vi "PAQmem_WriteOne.vi"(7 "Carry":bool, 8 "error in (no error)":errorcluster, 10 "StoreDatagram":T1 {"Time" format="%#.2f"; "status" format="%x"; "min" format="%.2f"; "max" format="%.2f"; "data" format="%.2f"}, 11 "PAQ-memory in":refnum<class "PAQ-memory.lvclass">) -> (0 "error out":errorcluster, 1 "Last":i32, 2 "Prev":i32, 3 "PAQ-memory out":refnum<class "PAQ-memory.lvclass">)   [LabVIEW 2020, in "Sgraph_lib_V1.lvlib" / "PAQ-memory.lvclass"]
doc: "PAQ memory action: write one sample (of multiple TAGs)\n\nThis VI writes one array of TAGs to the computer memory DVR element"
uses:
  PAQ-memory.lvclass
  controls/MemStoreDatagram.ctl
  PAQ-memory.lvclass/PAQ-memory.ctl
  FAMM.lvclass
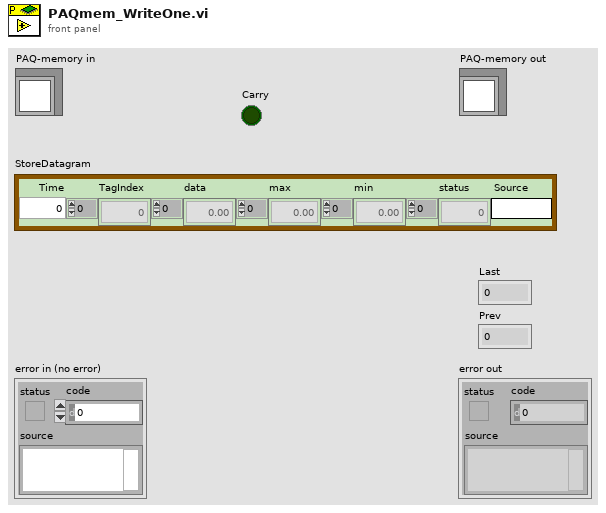
[diagram p1: front panel]
types:
  T1 = typedef "Sgraph_lib_V1.lvlib/FAMM.lvclass/MemStoreDatagram.ctl" = cluster{"Time":dbl, "TagIndex":i32[], "data":dbl[], "max":dbl[], "min":dbl[], "status":u32[], "Source":string}
  T2 = cluster{"source":refnum<data-value>, "status":refnum<data-value>, "data":refnum<data-value>, "max":refnum<data-value>, "min":refnum<data-value>}[]
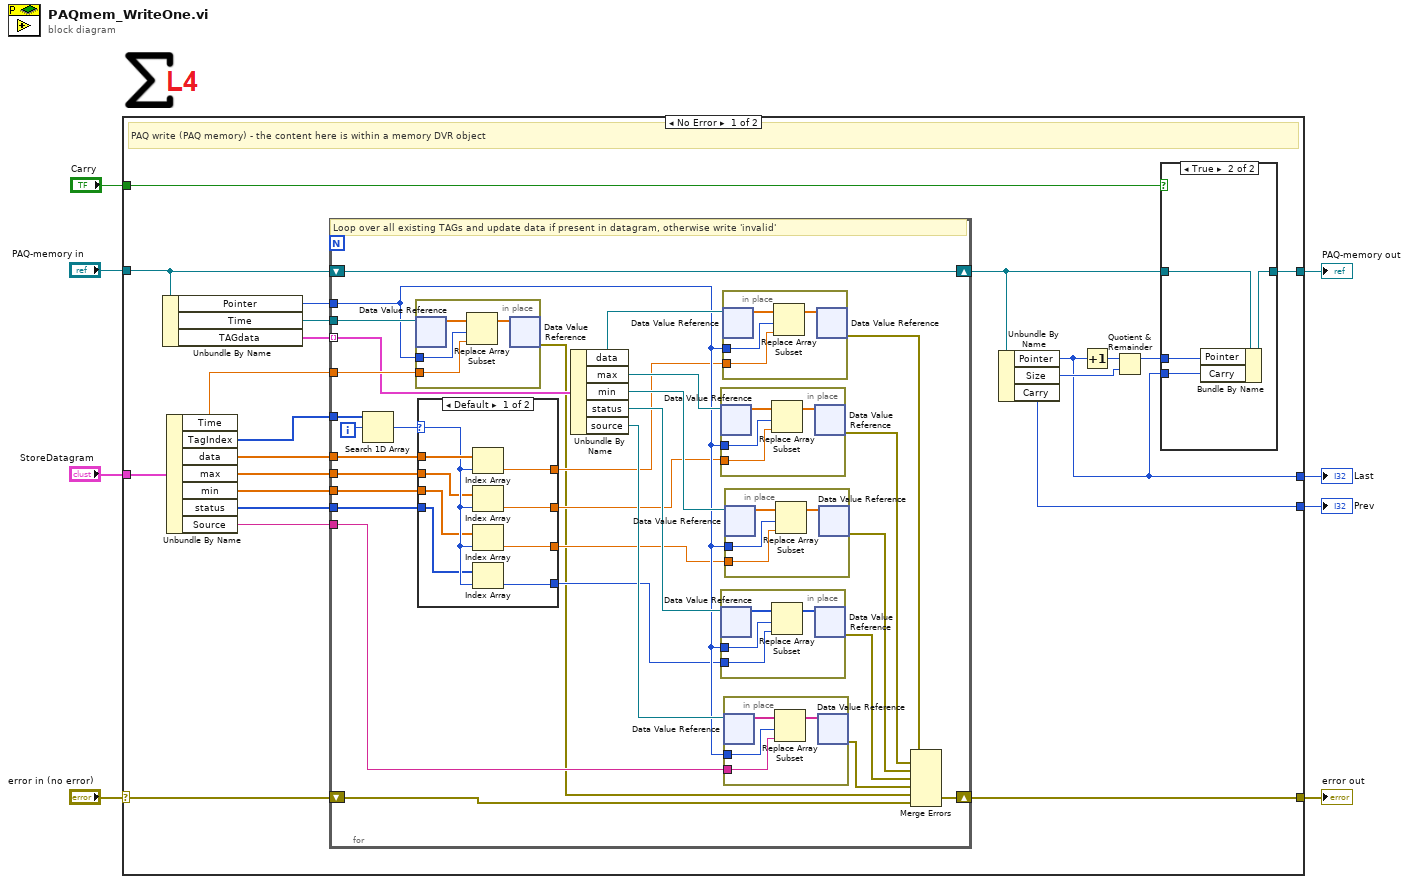
[diagram p0: block diagram]
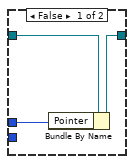
[diagram p2: hidden frame]
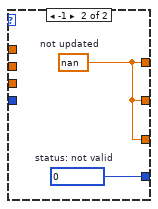
[diagram p3: hidden frame]
diagram:
  n1 = case shown="No Error" "error in (no error)" {
    selector: "error in (no error)" -> [w22 w104]
    tunnel: [w21 w104] -> w7
    tunnel: [w13 w103] -> w5
    tunnel: "PAQ-memory in" -> [w20 w103]
    tunnel: "StoreDatagram" -> [w30 _]
    tunnel: [w9 _] -> w3
    tunnel: "Carry" -> [w11 _]
    tunnel: [w10 _] -> w1
    frame No Error {
      # "PAQ write (PAQ memory) - the content here is within a memory DVR object"
      n2 = Unbundle By Name(w20) -> ("Pointer"=w19:i32, "Time"=w18:refnum<data-value>, "TAGdata"=w17:T2)
      n3 = Unbundle By Name(w30) -> ("Time"=w29:dbl, "TagIndex"=w28:i32[], "data"=w27:dbl[], "max"=w26:dbl[], "min"=w25:dbl[], "status"=w24:u32[], "Source"=w23:string)
      n4 = for {
        tunnel: w29 -> [w65]
        tunnel: w28 -> [w64]
        tunnel: w27 -> [w61]
        tunnel: w26 -> [w60]
        tunnel: w25 -> [w59]
        tunnel: w24 -> [w58]
        tunnel: w23 -> [w46]
        shift-right: [w43] -> w21
        shift-left: w22 -> [w45]
        shift-right: [w67] -> w14
        shift-left: w20 -> [w67]
        tunnel: w19 -> [w51]
        tunnel: w18 -> [w66]
        tunnel: w17 -> [w57] mode=indexing
        i -> [w63]
        # "Loop over all existing TAGs and update data if present in datagram, otherwise write 'invalid'"
        n5 = Search 1D Array(1D array=w64, element=w63) -> (index of element=w62:i32)  [unwired: 1 in]
        n6 = in-place {
          in-place-border: w51 -> [w100]
          in-place-border: w65 -> [w99]
          n7 = in-place-dvr #1(w66) -> (w102:dbl[])  [unwired: 1 out]
          n8 = Replace Array Subset(array=w102, new element=w99, index=w100) -> (w101:dbl[])
          n9 = in-place-dvr #1(w101) -> (w38:errorcluster)  [unwired: 1 out]
        }
        n10 = case shown="Default" w62 {
          selector: w62 -> [w95 _]
          tunnel: w61 -> [w96 _]
          tunnel: w60 -> [w94 _]
          tunnel: w59 -> [w93 _]
          tunnel: w58 -> [w92 _]
          tunnel: [w91 w98] -> w50
          tunnel: [w90 w98] -> w49
          tunnel: [w89 w98] -> w48
          tunnel: [w88 w97] -> w47
          frame Default {
            n11 = Index Array(array=w96, index=w95) -> (element=w91:dbl)
            n12 = Index Array(array=w94, index=w95) -> (element=w90:dbl)
            n13 = Index Array(array=w93, index=w95) -> (element=w89:dbl)
            n14 = Index Array(array=w92, index=w95) -> (element=w88:u32)
          }
          frame -1 {
            w97 = u32 0  # status: not valid
            w98 = nan  # not updated
          }
        }
        n15 = Unbundle By Name(w57) -> ("data"=w56:refnum<data-value>, "max"=w55:refnum<data-value>, "min"=w54:refnum<data-value>, "status"=w53:refnum<data-value>, "source"=w52:refnum<data-value>)
        n16 = in-place {
          in-place-border: w51 -> [w81]
          in-place-border: w49 -> [w80]
          n17 = in-place-dvr #2(w55) -> (w83:dbl[])  [unwired: 1 out]
          n18 = Replace Array Subset(array=w83, new element=w80, index=w81) -> (w82:dbl[])
          n19 = in-place-dvr #2(w82) -> (w42:errorcluster)  [unwired: 1 out]
        }
        n20 = in-place {
          in-place-border: w51 -> [w73]
          in-place-border: w47 -> [w72]
          n21 = in-place-dvr #3(w53) -> (w75:u32[])  [unwired: 1 out]
          n22 = Replace Array Subset(array=w75, new element=w72, index=w73) -> (w74:u32[])
          n23 = in-place-dvr #3(w74) -> (w40:errorcluster)  [unwired: 1 out]
        }
        n24 = in-place {
          in-place-border: w51 -> [w85]
          in-place-border: w50 -> [w84]
          n25 = in-place-dvr #4(w56) -> (w87:dbl[])  [unwired: 1 out]
          n26 = Replace Array Subset(array=w87, new element=w84, index=w85) -> (w86:dbl[])
          n27 = in-place-dvr #4(w86) -> (w44:errorcluster)  [unwired: 1 out]
        }
        n28 = in-place {
          in-place-border: w51 -> [w69]
          in-place-border: w46 -> [w68]
          n29 = in-place-dvr #5(w52) -> (w71:string[])  [unwired: 1 out]
          n30 = Replace Array Subset(array=w71, new element=w68, index=w69) -> (w70:string[])
          n31 = in-place-dvr #5(w70) -> (w39:errorcluster)  [unwired: 1 out]
        }
        n32 = in-place {
          in-place-border: w51 -> [w77]
          in-place-border: w48 -> [w76]
          n33 = in-place-dvr #6(w54) -> (w79:dbl[])  [unwired: 1 out]
          n34 = Replace Array Subset(array=w79, new element=w76, index=w77) -> (w78:dbl[])
          n35 = in-place-dvr #6(w78) -> (w41:errorcluster)  [unwired: 1 out]
        }
        n36 = Merge Errors(w44, w42, w41, w40, w39, w38, w45) -> (w43:errorcluster)
      }
      n37 = Unbundle By Name(w14) -> ("Pointer"=w9:i32, "Size"=w15:i32, "Carry"=w10:i32)
      n38 = Increment(x=w9) -> (x+1=w16:i32)
      n39 = Quotient & Remainder(x=w16, y=w15) -> (x-y*floor(x/y)=w12:i32)  [unwired: 1 out]
      n40 = case shown="True" w11 {
        tunnel: w14 -> [w33 w37]
        tunnel: [w32 w36] -> w13
        tunnel: w12 -> [w31 w35]
        tunnel: w9 -> [_ w34]
        frame False {
          n41 = Bundle By Name(cluster=w33, "Pointer"=w31) -> (w32:refnum<class "PAQ-memory.lvclass">)
        }
        frame True {
          n42 = Bundle By Name(cluster=w37, "Pointer"=w35, "Carry"=w34) -> (w36:refnum<class "PAQ-memory.lvclass">)
        }
      }
    }
    frame Error {
    }
  }
  "error out" <- w7
  "PAQ-memory out" <- w5
  "Last" <- w3
  "Prev" <- w1
